vi "ziGetEventByteArray.vi"(8 "Error In":errorcluster, 10 "ByteArray In":T1, 11 "Handle In":T2 {"Handle" format="0x%08x"; "Conn" format="0x%08x"}) -> (0 "Error Out":errorcluster, 2 "ByteArray Out":T1, 3 "Handle Out":T2 {"Handle" format="0x%08x"; "Conn" format="0x%08x"})   [LabVIEW 2009, in "Zurich Instruments LabOne.lvlib"]
uses:
  <instrlib>/Zurich Instruments LabOne/Zurich Instruments LabOne.lvlib
  <instrlib>/Zurich Instruments LabOne/Public/ziTypeHandle.ctl
  <instrlib>/Zurich Instruments LabOne/Public/Data/ziTypeByteArray.ctl
  <instrlib>/Zurich Instruments LabOne/Private/ziLV32.dll
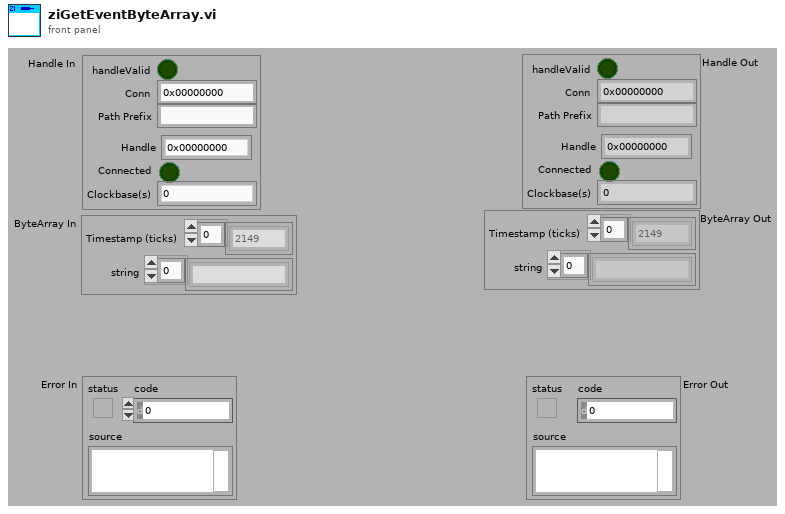
[diagram p1: front panel]
types:
  T1 = typedef "Zurich Instruments LabOne.lvlib/ziTypeByteArray.ctl" = cluster{"Timestamp (ticks)":u64[], "string":string[]}
  T2 = typedef "Zurich Instruments LabOne.lvlib/ziTypeHandle.ctl" = cluster{"handleValid":bool, "Conn":u64, "Path Prefix":string, "Handle":u64, "Connected":bool, "Clockbase(s)":dbl}
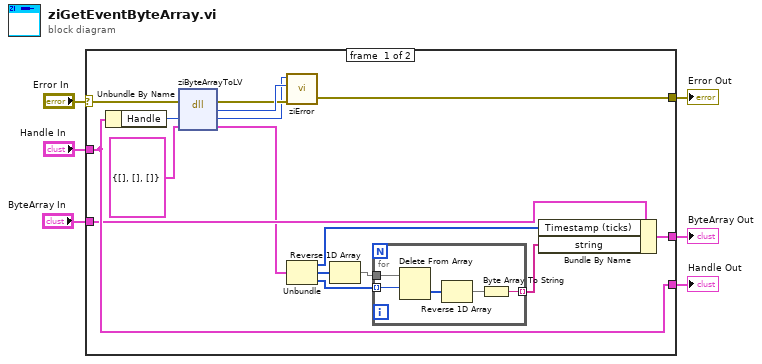
[diagram p0: block diagram]
diagram:
  n1 = case shown="No Error" "Error In" {
    selector: "Error In" -> [w21 w30]
    tunnel: "Handle In" -> [w17 w28]
    tunnel: [w17 w28] -> w5
    tunnel: [w13 w29] -> w4
    tunnel: "ByteArray In" -> [w14 w29]
    tunnel: [w22 w30] -> w2
    frame #0 {
      n2 = Unbundle By Name(w17) -> ("Handle"=w19:u64)
      n3 = dll-call lib="C:/Program Files (x86)/National Instruments/LabVIEW 2009/instr.lib/Zurich Instruments LabOne/Private/ziLV*.*" fn="ziByteArrayToLV"(error in=w21, "ziEventBuffer"=w19, cluster{u64[], u8[], u64[]} {[], [], []}) -> (error out=w18:errorcluster, "return type"=w20:u32, "ziEventBuffer"=w16:u64, w12:cluster{u64[], u8[], u64[]})  [unwired: 2 in, 1 out]
      n4 = call <instrlib>:"ziError.vi"("Conn"=w16, "ziErrorCode"=w20, "Error In"=w18) -> ("Error Out"=w22:errorcluster)  [unwired: 2 in, 1 out]
      n5 = Unbundle(w12) -> (w7:u64[], w8:u8[], w11:u64[])
      n6 = Reverse 1D Array(array=w8) -> (reversed array=w10:u8[])
      n7 = for {
        tunnel: w11 -> [w25] mode=indexing
        tunnel: w10 -> [w26]
        tunnel: [w27] -> w9 mode=indexing
        n8 = Delete From Array(array=w26, length=w25) -> (deleted portion=w24:u8[])  [unwired: 1 in, 1 out]
        n9 = Reverse 1D Array(array=w24) -> (reversed array=w23:u8[])
        n10 = Byte Array To String(unsigned byte array=w23) -> (string=w27:string)
      }
      n11 = Bundle By Name(cluster=w14, "Timestamp (ticks)"=w7, "string"=w9) -> (w13:T1)
    }
    frame #1 {
    }
  }
  "Handle Out" <- w5
  "ByteArray Out" <- w4
  "Error Out" <- w2
